vi "RH Tester.vi"() -> ()   [LabVIEW 2011]
uses:
  <vilib>/Platform/TimedLoop/XDataNode/timing_clust.ctl
  <vilib>/Platform/TimedLoop/XDataNode/nitl_modes.ctl
  <vilib>/Platform/TimedLoop/XDataNode/wakeup.ctl
  <vilib>/Utility/file.llb/Write To Spreadsheet File (string).vi
  <vilib>/Platform/TimedLoop/XDataNode/XDataNode.xnode
  <vilib>/Platform/TimedLoop/XDataNode/XDNodeRunTimeDep.lvlib
panel:
  out "Probe 2 RH":dbl
  out "Probe 2 (F)":dbl
  out "Probe 2 Error":errorcluster
  in  "Probe 2":string="192.168.1.42"
  out "Probe 1 RH":dbl
  out "Probe 1 (F)":dbl
  in  "Probe 1":string="192.168.1.41"
  in  "Chamber Temp":string="192.168.1.161"
  out "Probe 1 Error":errorcluster
  out "Chamber Temp Error":errorcluster
  in  "Log Data":bool=TRUE
  out "RH":cluster{dbl[], dbl[]}[](graph)
  in  "Period(s)":i32=10
  in  "Max Num to Chart":i32=1000
  out "Temp":cluster{dbl[], dbl[]}[](graph)
  out "Chamber RH":dbl
  out "Chamber Temp (F)":dbl
  out "time stamp":timestamp
  out "Count":i32
  in  "stop":bool
  in  "file path (dialog if empty)":path=path "c:/data/RH_Log_Data.csv"
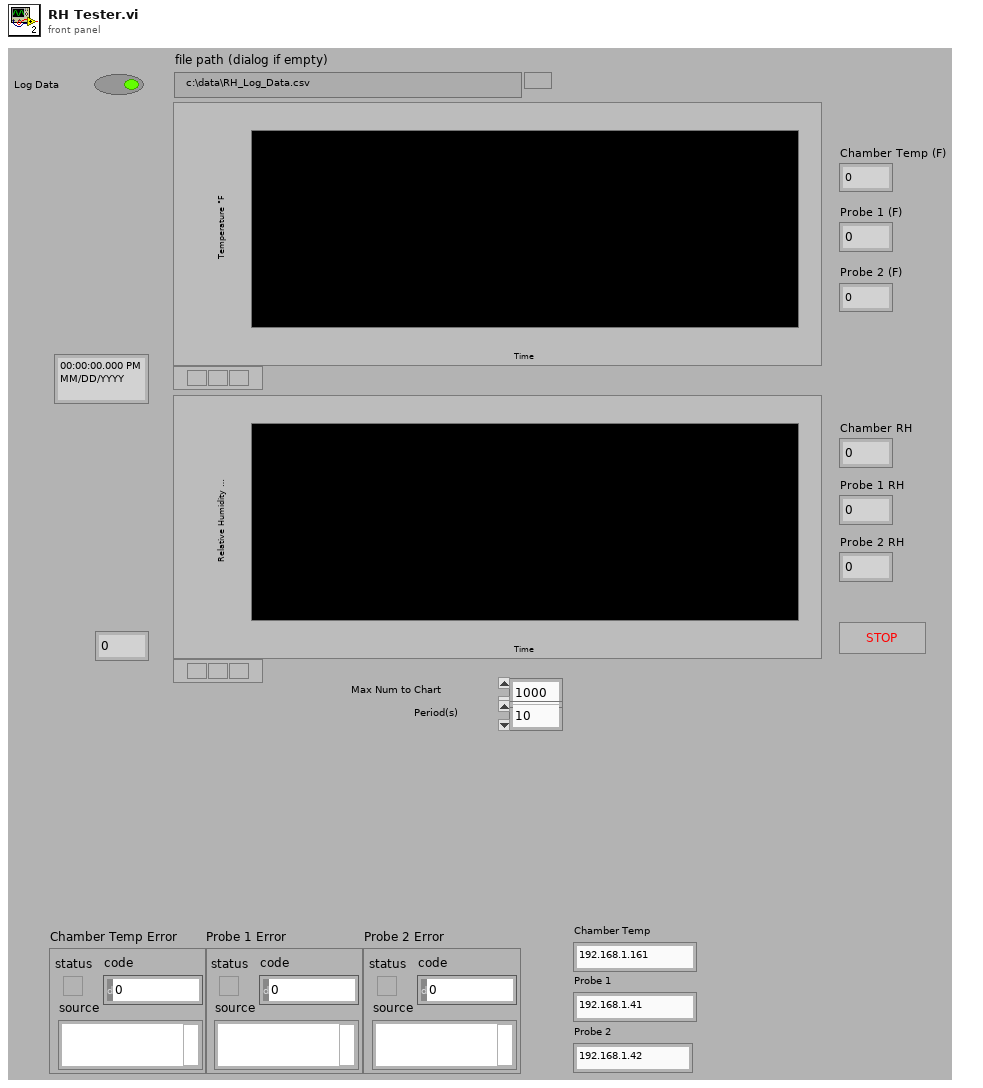
[diagram p1: front panel]
types:
  T1 = typedef "XDNodeRunTimeDep.lvlib/timing_clust.ctl" = cluster{"Expected End [f-1]":u64, "Actual End [f-1]":u64, "Finished Late? [f-1]":bool, "Expected End [i-1]":u64, "Actual End [i-1]":u64, "Finished Late? [i-1]":bool, "Expected Start [i]":u64, "Actual Start [i]":u64, "Expected Start [f]":u64, "Actual Start [f]":u64, "Source Name":string, "Structure Name":string, "Period":i64, "Deadline":i64, "Offset":i64, "Start":i64, "Priority":i32, "Timeout":i32, "Mode":T2, "Wakeup Reason":T3, "Error":errorcluster, "Source Type":string, "Secondary Source Type":string, "Global End Time":u64, "Global Start Time":u64, "Frame Duration":u64, "Iteration Duration":u64, "Assigned CPU":i32, "I/O Scan Engine Mode":u32}
  T2 = typedef "XDNodeRunTimeDep.lvlib/nitl_modes.ctl" = enum32{"No Change", "Process missed periods, maintain original phase", "Discard missed periods, maintain original phase", "Process missed periods, ignore original phase", "Discard missed periods, ignore original phase"}
  T3 = typedef "XDNodeRunTimeDep.lvlib/wakeup.ctl" = enum32{"Normal", "Aborted", "Asynchronous wakeup", "Timing source error", "Timed loop error", "Timeout"}
  T4 = cluster{"[Temp (F), RH][0]":dbl, "[Temp (F), RH][1]":dbl}
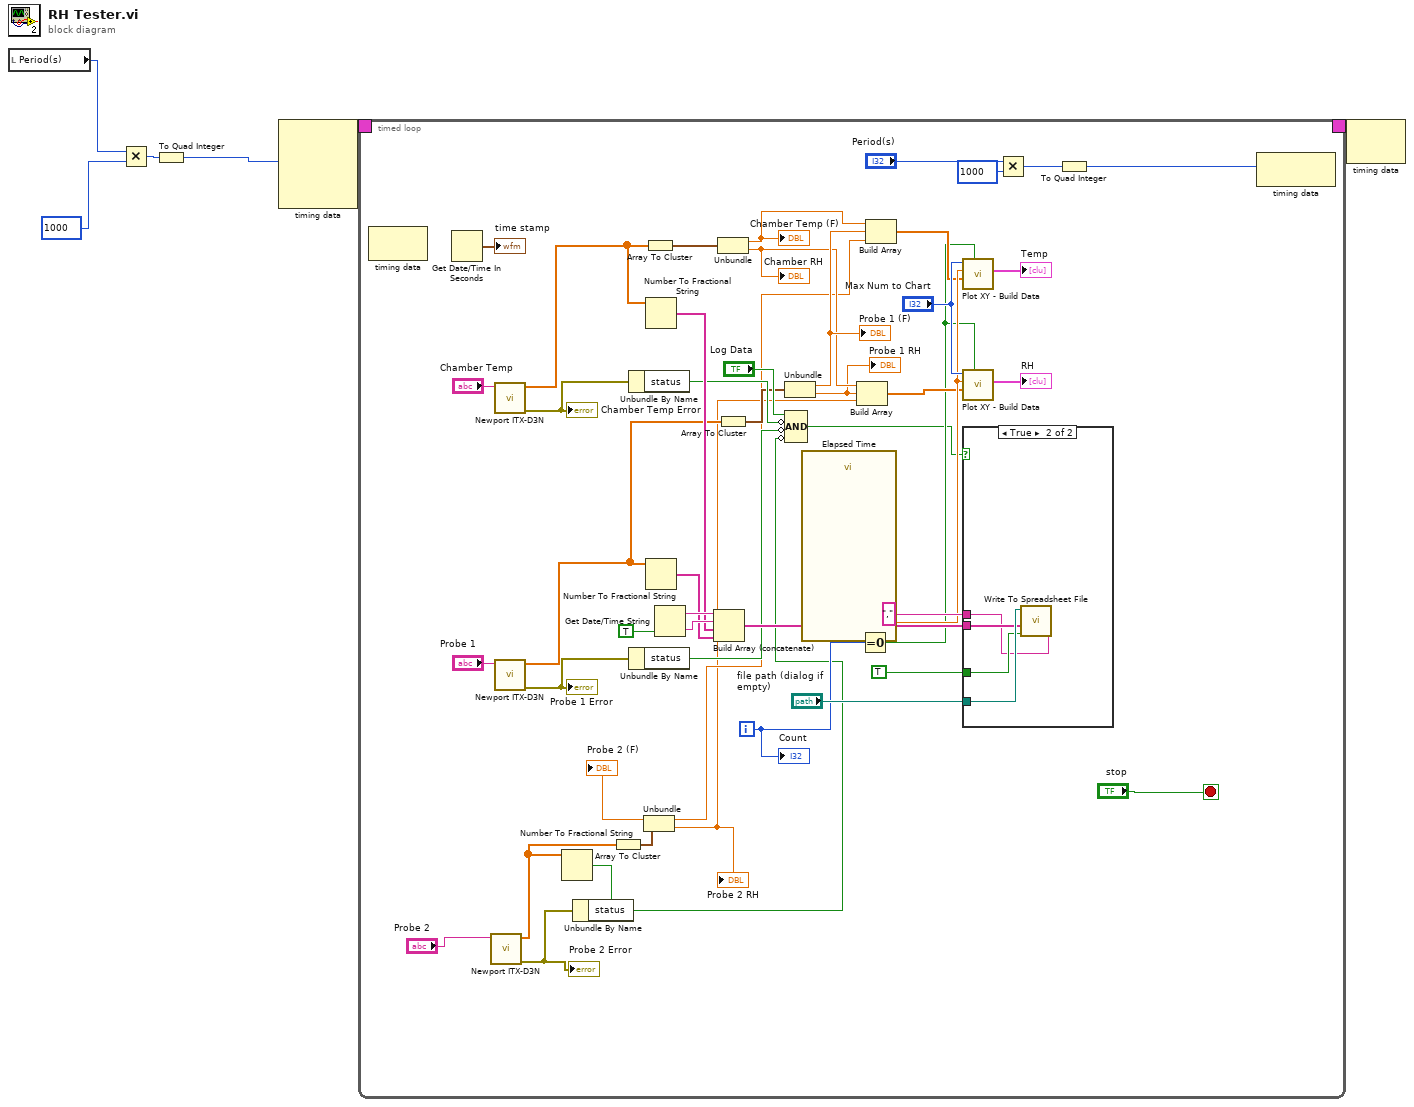
[diagram p0: block diagram]
diagram:
  n1 = local read "Period(s)"() -> (w1:i32)
  n2 = Multiply(x=w1, y=1000) -> (x*y=w3:i32)
  n3 = To Quad Integer(1:w3) -> (0:w2:i64)
  n4 = node-c288(w2) -> (w6:T1)  [unwired: 3 in]
  n5 = timed-loop {
    timing: w6 -> [_]
    timing-out: [_] -> w5
    i -> [w31]
    stop <- "stop" stop-if-true
    n6 = node-c288() -> ()  [unwired: 1 in, 1 out]
    n7 = Get Date/Time In Seconds() -> (seconds since 1Jan1904=→"time stamp":timestamp)
    n8 = call "Newport ITX-D3N.vi"("Machine"="Probe 2") -> ("error out"=w12:errorcluster, "[Temp (F), RH]"=w10:dbl[])  [unwired: 9 in]
    "Probe 2 Error" <- w12
    n9 = call "Newport ITX-D3N.vi"("Machine"="Chamber Temp") -> ("error out"=w24:errorcluster, "[Temp (F), RH]"=w39:dbl[])  [unwired: 9 in]
    "Chamber Temp Error" <- w24
    n10 = call "Newport ITX-D3N.vi"("Machine"="Probe 1") -> ("error out"=w20:errorcluster, "[Temp (F), RH]"=w17:dbl[])  [unwired: 9 in]
    "Probe 1 Error" <- w20
    n11 = Unbundle By Name(w12) -> ("status"=w11:bool)
    n12 = Number To Fractional String(use system decimal point (T)=w11, number=w10) -> ()  [unwired: 2 in, 1 out]
    n13 = Array To Cluster(array=w10) -> (cluster=w9:T4)
    n14 = Unbundle By Name(w24) -> ("status"=w23:bool)
    n15 = Unbundle By Name(w20) -> ("status"=w19:bool)
    n16 = Unbundle(w9) -> ("[Temp (F), RH][0]"=w8:dbl, "[Temp (F), RH][1]"=w7:dbl)
    "Probe 2 (F)" <- w8
    "Probe 2 RH" <- w7
    n17 = Array To Cluster(array=w39) -> (cluster=w42:T4)
    n18 = Number To Fractional String(number=w39) -> (F-format string=w48:string[])  [unwired: 3 in]
    n19 = Number To Fractional String(number=w17) -> (F-format string=w21:string[])  [unwired: 3 in]
    n20 = Get Date/Time String(want seconds? (F)=TRUE) -> (date string=w50:string, time string=w49:string)  [unwired: 2 in]
    n21 = Build Array (concatenate)(w50, w49, w48, w21) -> (w46:string[])
    n22 = Unbundle(w42) -> ("[Temp (F), RH][0]"=w33:dbl, "[Temp (F), RH][1]"=w15:dbl)
    "Chamber Temp (F)" <- w33
    "Chamber RH" <- w15
    n23 = Array To Cluster(array=w17) -> (cluster=w18:T4)
    n24 = Unbundle(w18) -> ("[Temp (F), RH][0]"=w16:dbl, "[Temp (F), RH][1]"=w14:dbl)
    "Probe 1 (F)" <- w16
    "Probe 1 RH" <- w14
    n25 = Compound Arithmetic op=AND("Log Data", invert w23, invert w19, invert w11) -> (w25:bool)
    n26 = call "Elapsed Time"() -> ("Present (s)"=w36:dbl)  [unwired: 12 in, 7 out]
    n27 = Build Array(w15, w14, w7) -> (w35:dbl[])
    n28 = Equal To 0?(x=w31) -> (x = 0?=w30:bool)
    n29 = Build Array(w33, w16, w8) -> (w34:dbl[])
    n30 = call "Plot XY - Build Data.vi"("Reset"=w30, "Data Array"=w34, "Time (s)"=w36, "Max Array Size"="Max Num to Chart") -> ("Plot Data"=→"Temp":cluster{dbl[], dbl[]}[])  [unwired: 7 in]
    n31 = call "Plot XY - Build Data.vi"("Reset"=w30, "Data Array"=w35, "Time (s)"=w36, "Max Array Size"="Max Num to Chart") -> ("Plot Data"=→"RH":cluster{dbl[], dbl[]}[])  [unwired: 7 in]
    n32 = case shown="True" w25 {
      tunnel: "file path (dialog if empty)" -> [_ w56]
      tunnel: w46 -> [_ w55]
      tunnel: TRUE ("append to file? (new file:F)") -> [_ w54]
      tunnel: "," ("delimiter (\\t)") -> [_ w53]
      frame False {
      }
      frame True {
        n33 = call-poly <vilib>:"Write To Spreadsheet File.vi"("delimiter (\\t)"=w53, "append to file? (new file:F)"=w54, "1D data"=w55, "file path (dialog if empty)"=w56) -> ()  [unwired: 4 in, 1 out]
      }
    }
    n34 = Multiply(x="Period(s)", y=1000) -> (x*y=w29:i32)
    n35 = To Quad Integer(1:w29) -> (0:w27:i64)
    n36 = node-c288(w27) -> ()  [unwired: 1 out]
    "Count" <- w31
  }
  n37 = node-c288(w5) -> ()  [unwired: 1 out]
